vi "DAQ Init_New.vi"(11 "Model":string) -> (0 "Task_Hall_5":refnum<k21>, 1 "Task_Resistors":refnum<k21>, 2 "Task_Hall_1":refnum<k21>, 3 "Task_Capacitor":refnum<k21>, 4 "Task_Hall_3":refnum<k21>, 5 "Task_Hall_2":refnum<k21>, 6 "Task_Crash_Signal":refnum<k21>, 7 "Task_Passive_Lock":refnum<k21>, 8 "Task_OHS":refnum<k21>, 9 "Task_Hall_4":refnum<k21>, 10 "Task_IBH_Switch":refnum<k21>)   [LabVIEW 2023]
uses:
  <vilib>/DAQmx/create/channels.llb/DAQmx Create Channel (DO-Digital Output).vi
panel:
  out "error out":errorcluster
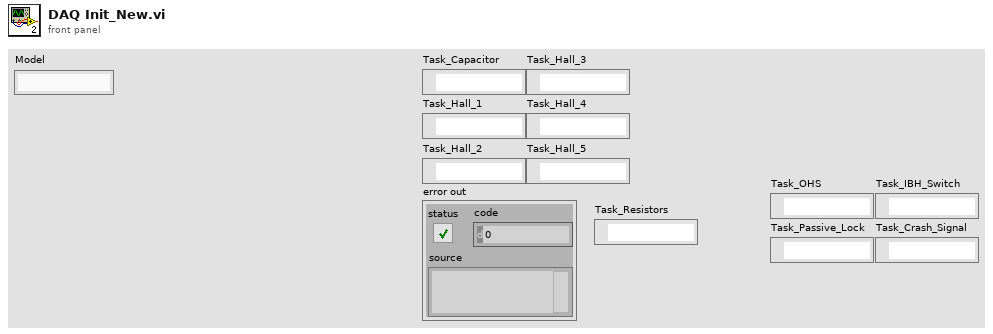
[diagram p1: front panel]
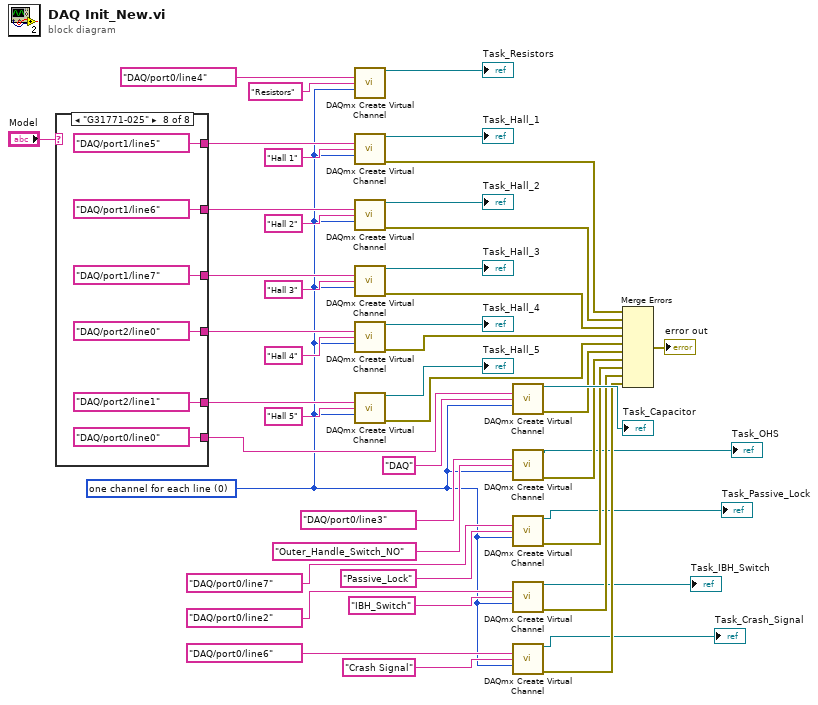
[diagram p0: block diagram]
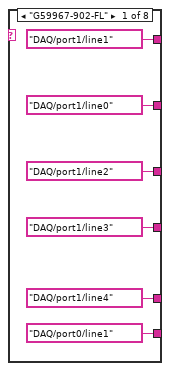
[diagram p2: hidden frame]
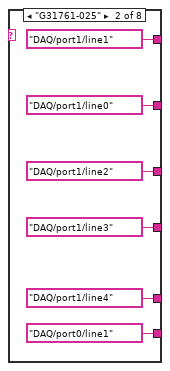
[diagram p3: hidden frame]
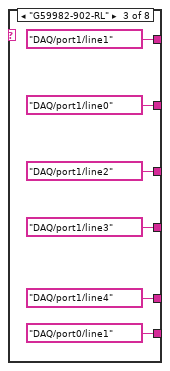
[diagram p4: hidden frame]
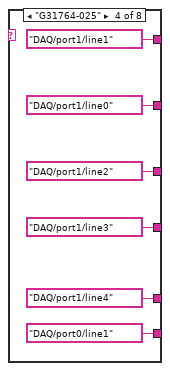
[diagram p5: hidden frame]
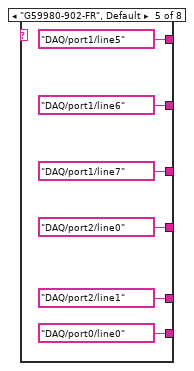
[diagram p6: hidden frame]
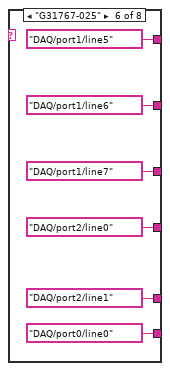
[diagram p7: hidden frame]
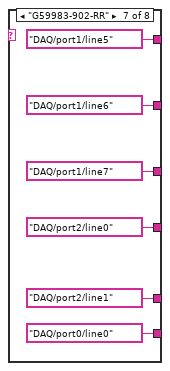
[diagram p8: hidden frame]
diagram:
  w9 = 0 items=["one channel for each line", "one channel for all lines"] ("line grouping")
  n1 = case shown="\"G31771-025\"" "Model" {
    tunnel: [tag "DAQ/port0/line1" ("lines") tag "DAQ/port0/line1" ("lines") tag "DAQ/port0/line1" ("lines") tag "DAQ/port0/line1" ("lines") tag "DAQ/port0/line0" ("lines") tag "DAQ/port0/line0" ("lines") tag "DAQ/port0/line0" ("lines") tag "DAQ/port0/line0" ("lines")] -> w44
    tunnel: [tag "DAQ/port1/line4" ("lines") tag "DAQ/port1/line4" ("lines") tag "DAQ/port1/line4" ("lines") tag "DAQ/port1/line4" ("lines") tag "DAQ/port2/line1" ("lines") tag "DAQ/port2/line1" ("lines") tag "DAQ/port2/line1" ("lines") tag "DAQ/port2/line1" ("lines")] -> w37
    tunnel: [tag "DAQ/port1/line3" ("lines") tag "DAQ/port1/line3" ("lines") tag "DAQ/port1/line3" ("lines") tag "DAQ/port1/line3" ("lines") tag "DAQ/port2/line0" ("lines") tag "DAQ/port2/line0" ("lines") tag "DAQ/port2/line0" ("lines") tag "DAQ/port2/line0" ("lines")] -> w36
    tunnel: [tag "DAQ/port1/line2" ("lines") tag "DAQ/port1/line2" ("lines") tag "DAQ/port1/line2" ("lines") tag "DAQ/port1/line2" ("lines") tag "DAQ/port1/line7" ("lines") tag "DAQ/port1/line7" ("lines") tag "DAQ/port1/line7" ("lines") tag "DAQ/port1/line7" ("lines")] -> w35
    tunnel: [tag "DAQ/port1/line1" ("lines") tag "DAQ/port1/line1" ("lines") tag "DAQ/port1/line1" ("lines") tag "DAQ/port1/line1" ("lines") tag "DAQ/port1/line5" ("lines") tag "DAQ/port1/line5" ("lines") tag "DAQ/port1/line5" ("lines") tag "DAQ/port1/line5" ("lines")] -> w34
    tunnel: [tag "DAQ/port1/line0" ("lines") tag "DAQ/port1/line0" ("lines") tag "DAQ/port1/line0" ("lines") tag "DAQ/port1/line0" ("lines") tag "DAQ/port1/line6" ("lines") tag "DAQ/port1/line6" ("lines") tag "DAQ/port1/line6" ("lines") tag "DAQ/port1/line6" ("lines")] -> w33
    frame "G59967-902-FL" {
    }
    frame "G31761-025" {
    }
    frame "G59982-902-RL" {
    }
    frame "G31764-025" {
    }
    frame "G59980-902-FR", Default {
    }
    frame "G31767-025" {
    }
    frame "G59983-902-RR" {
    }
    frame "G31771-025" {
    }
  }
  n2 = call-poly <vilib>:"DAQmx Create Virtual Channel.vi"("lines"=tag "DAQ/port0/line4", "name to assign"="Resistors", "line grouping"=w9) -> ("task out"=→"Task_Resistors":refnum<k21>)  [unwired: 11 in, 1 out]
  n3 = call-poly <vilib>:"DAQmx Create Virtual Channel.vi"("lines"=w34, "name to assign"="Hall 1", "line grouping"=w9) -> ("task out"=→"Task_Hall_1":refnum<k21>, "error out"=w27:errorcluster)  [unwired: 11 in]
  n4 = call-poly <vilib>:"DAQmx Create Virtual Channel.vi"("lines"=w33, "name to assign"="Hall 2", "line grouping"=w9) -> ("task out"=→"Task_Hall_2":refnum<k21>, "error out"=w26:errorcluster)  [unwired: 11 in]
  n5 = call-poly <vilib>:"DAQmx Create Virtual Channel.vi"("lines"=w35, "name to assign"="Hall 3", "line grouping"=w9) -> ("task out"=→"Task_Hall_3":refnum<k21>, "error out"=w25:errorcluster)  [unwired: 11 in]
  n6 = call-poly <vilib>:"DAQmx Create Virtual Channel.vi"("lines"=w36, "name to assign"="Hall 4", "line grouping"=w9) -> ("task out"=→"Task_Hall_4":refnum<k21>, "error out"=w24:errorcluster)  [unwired: 11 in]
  n7 = call-poly <vilib>:"DAQmx Create Virtual Channel.vi"("lines"=w37, "name to assign"="Hall 5", "line grouping"=w9) -> ("task out"=→"Task_Hall_5":refnum<k21>, "error out"=w23:errorcluster)  [unwired: 11 in]
  n8 = call-poly <vilib>:"DAQmx Create Virtual Channel.vi"("lines"=w44, "name to assign"="DAQ", "line grouping"=w9) -> ("task out"=→"Task_Capacitor":refnum<k21>, "error out"=w22:errorcluster)  [unwired: 11 in]
  n9 = call-poly <vilib>:"DAQmx Create Virtual Channel.vi"("lines"=tag "DAQ/port0/line3", "name to assign"="Outer_Handle_Switch_NO", "line grouping"=w9) -> ("task out"=→"Task_OHS":refnum<k21>, "error out"=w8:errorcluster)  [unwired: 11 in]
  n10 = call-poly <vilib>:"DAQmx Create Virtual Channel.vi"("lines"=tag "DAQ/port0/line7", "name to assign"="Passive_Lock", "line grouping"=w9) -> ("task out"=→"Task_Passive_Lock":refnum<k21>, "error out"=w7:errorcluster)  [unwired: 11 in]
  n11 = call-poly <vilib>:"DAQmx Create Virtual Channel.vi"("lines"=tag "DAQ/port0/line2", "name to assign"="IBH_Switch", "line grouping"=w9) -> ("task out"=→"Task_IBH_Switch":refnum<k21>, "error out"=w6:errorcluster)  [unwired: 11 in]
  n12 = call-poly <vilib>:"DAQmx Create Virtual Channel.vi"("lines"=tag "DAQ/port0/line6", "name to assign"="Crash Signal", "line grouping"=w9) -> ("task out"=→"Task_Crash_Signal":refnum<k21>, "error out"=w5:errorcluster)  [unwired: 11 in]
  n13 = Merge Errors(w27, w26, w25, w24, w23, w22, w8, w7, w6, w5) -> (→"error out":errorcluster)
